vi "Restore Moved Files.vi"(8 "error in (no error)":errorcluster, 11 "Builder in":refnum<class "Builder.lvclass">) -> (0 "error out":errorcluster, 3 "Builder out":refnum<class "Builder.lvclass">)   [LabVIEW 2019, in "Builder.lvclass"]
uses:
  Builder/Builder.lvclass
  Builder/Builder.lvclass/Builder.ctl
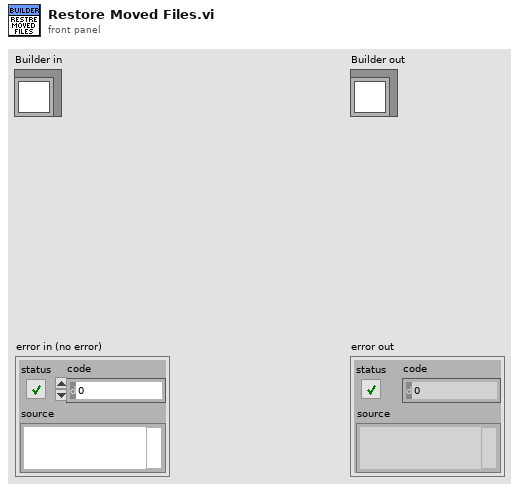
[diagram p1: front panel]
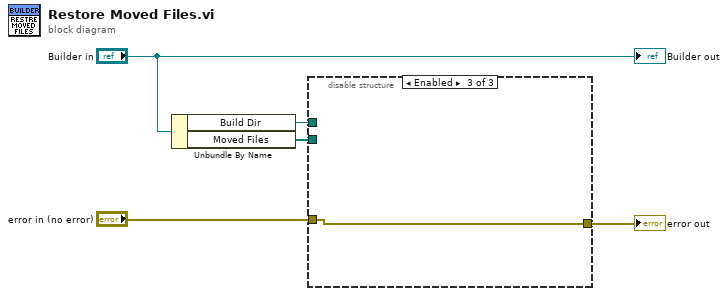
[diagram p0: block diagram]
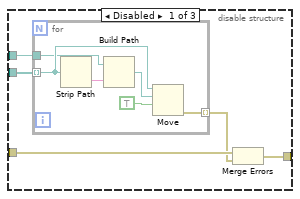
[diagram p2: hidden frame]
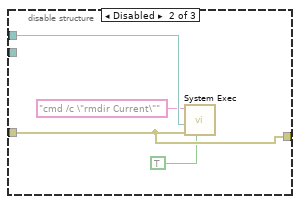
[diagram p3: hidden frame]
diagram:
  n1 = Unbundle By Name("Builder in") -> ("Build Dir"=w2:path, "Moved Files"=w1:path[])
  n2 = disable-structure shown="Enabled" {
    disable-tunnel: "error in (no error)" -> [w10 w18 w21]
    disable-tunnel: [w8 w18 w21] -> w4
    disable-tunnel: w2 -> [w7 w20 _]
    disable-tunnel: w1 -> [w6 _ _]
    frame Disabled {
      n3 = for {
        tunnel: w7 -> [w12]
        tunnel: w6 -> [w14] mode=indexing
        tunnel: [w16] -> w9 mode=indexing
        n4 = Strip Path(path=w14) -> (name=w13:string)  [unwired: 1 out]
        n5 = Build Path(base path=w12, name or relative path=w13) -> (appended path=w11:path)
        n6 = Move(source path=w14, 9:TRUE ("overwrite (F)"), 10:w11) -> (error out=w16:errorcluster)  [unwired: 2 in, 2 out]
      }
      n7 = Merge Errors(w10, w9) -> (w8:errorcluster)
    }
    frame Disabled {
      n8 = call <vilib>:"System Exec.vi"("run minimized? (F)"=TRUE, "error in (no error)"=w18, "working directory"=w20, "command line"="cmd /c \"rmdir Current\"") -> ()  [unwired: 4 in, 4 out]
    }
    frame Enabled {
    }
  }
  "error out" <- w4
  "Builder out" <- "Builder in"
